vi "BGP - Data - Stop.vi"(8 "error in (no error)":errorcluster) -> (0 "error out":errorcluster)   [LabVIEW 2012]
uses:
  Controls/Object Ref and Name.ctl
  Controls/Global Stop States.ctl
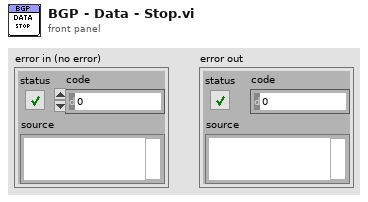
[diagram p1: front panel]
types:
  T1 = typedef "Object Ref and Name.ctl" = cluster{"Name":string, "Reference":refnum<vi>}
  T2 = typedef "Global Stop States.ctl" = enum16{"STOP", "STATUS", "INIT"}
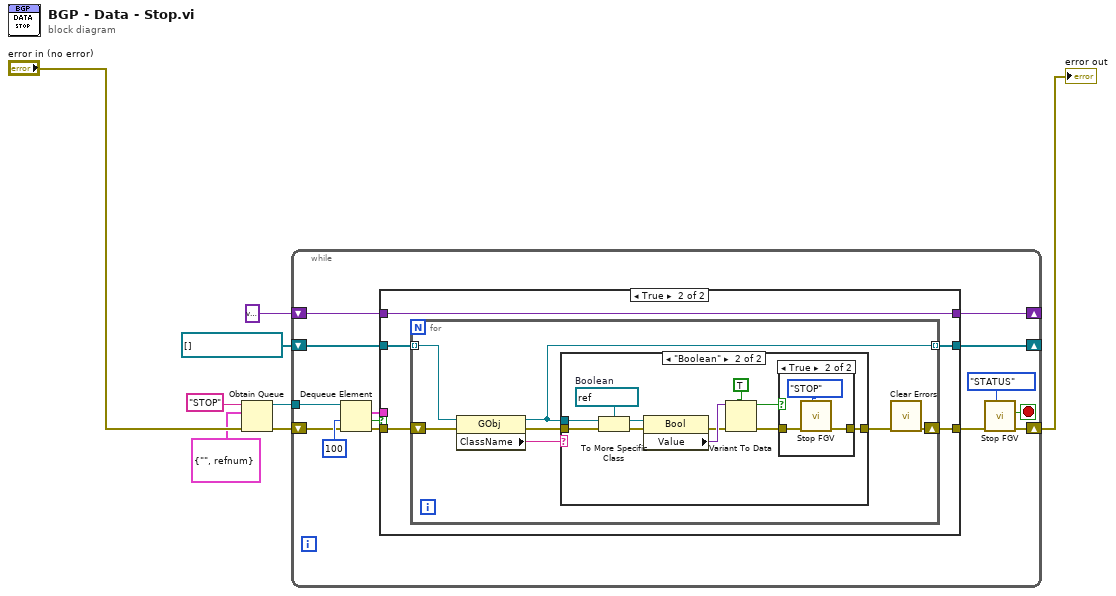
[diagram p0: block diagram]
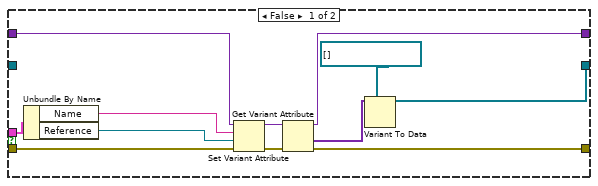
[diagram p2: hidden frame]
diagram:
  n1 = Obtain Queue(name (unnamed)="STOP", element data type=T1 {"Name"="", "Reference"=refnum}, error in (no error)="error in (no error)") -> (queue out=w6:refnum<queue>, error out=w2:errorcluster)  [unwired: 2 in, 1 out]
  n2 = while {
    tunnel: w6 -> [w22]
    shift-right: [w18] -> _
    shift-left: variant ("variant") -> [w20]
    shift-right: [w11] -> w7
    shift-left: w2 -> [w16]
    shift-right: [w15] -> _
    shift-left: refnum<vi>[] [] -> [w14]
    stop <- w9 stop-if-true
    n3 = Dequeue Element(queue=w22, timeout in ms (-1)=100, error in (no error)=w16) -> (element=w19:T1, timed out?=w13:bool, error out=w17:errorcluster)  [unwired: 1 out]
    n4 = case shown="True" w13 {
      tunnel: w20 -> [w34 w39]
      tunnel: w19 -> [w33 _]
      tunnel: [w29 w39] -> w18
      tunnel: w17 -> [w28 w38]
      tunnel: [w26 w35] -> w12
      tunnel: [w23 w36] -> w15
      tunnel: w14 -> [_ w37]
      frame False {
        n5 = Unbundle By Name(w33) -> ("Name"=w32:string, "Reference"=w31:refnum<vi>)
        n6 = Set Variant Attribute(Variant=w34, name=w32, value=w31, error in=w28) -> (Variant out=w30:variant, error out=w27:errorcluster)  [unwired: 1 out]
        n7 = Get Variant Attribute(Variant=w30, error in=w27) -> (duplicate Variant=w29:variant, values=w24:variant[], error out=w26:errorcluster)  [unwired: 2 in, 1 out]
        n8 = Variant To Data(type=refnum<vi>[] [], Variant=w24) -> (data=w23:refnum<vi>[])  [unwired: 1 in, 1 out]
      }
      frame True {
        n9 = for {
          tunnel: w37 -> [w46] mode=indexing
          shift-right: [w42] -> w35
          shift-left: w38 -> [w44]
          tunnel: [w45] -> w36 mode=indexing
          n10 = property class="GObj"(reference=w46, error in=w44) -> (reference out=w45:refnum<vi>, error out=w43:errorcluster, "ClassName"=w41:string)
          n11 = case shown="\"Boolean\"" w41 {
            tunnel: w45 -> [_ w56]
            tunnel: w43 -> [w47 w55]
            tunnel: [w47 w49] -> w40
            frame "False", Default {
            }
            frame "Boolean" {
              w58 = refnum<vi> refnum  # Boolean
              n12 = To More Specific Class(target class=w58, reference=w56, error in=w55) -> (specific class reference=w57:refnum<vi>, error out=w54:errorcluster)
              n13 = property class="Bool"(reference=w57, error in=w54) -> (error out=w52:errorcluster, "Value"=w53:variant)  [unwired: 1 out]
              n14 = Variant To Data(error in=w52, type=TRUE, Variant=w53) -> (data=w48:bool, error out=w50:errorcluster)
              n15 = case shown="True" w48 {
                tunnel: w50 -> [w59 w61]
                tunnel: [w59 w60] -> w49
                frame False {
                }
                frame True {
                  n16 = call "Stop FGV.vi"("Operation In"=Global_Stop_States."STOP", "error in"=w61) -> ("error out"=w60:errorcluster)  [unwired: 8 in, 1 out]
                }
              }
            }
          }
          n17 = call <vilib>:"Clear Errors.vi"("error in (no error)"=w40) -> ("error out"=w42:errorcluster)  [unwired: 6 in]
        }
      }
    }
    n18 = call "Stop FGV.vi"("Operation In"=Global_Stop_States."STATUS", "error in"=w12) -> ("error out"=w11:errorcluster, "Stop?"=w9:bool)  [unwired: 8 in]
  }
  "error out" <- w7
